vi "Add Point.vi"(8 "error in (no error)":errorcluster, 9 "Y":dbl, 10 "X":dbl, 11 "IV_data in":refnum<class "IV_data.lvclass">) -> (0 "error out":errorcluster, 3 "IV_data out":refnum<class "IV_data.lvclass">)   [LabVIEW 2014, in "IV_data.lvclass"]
uses:
  IV_data.lvclass
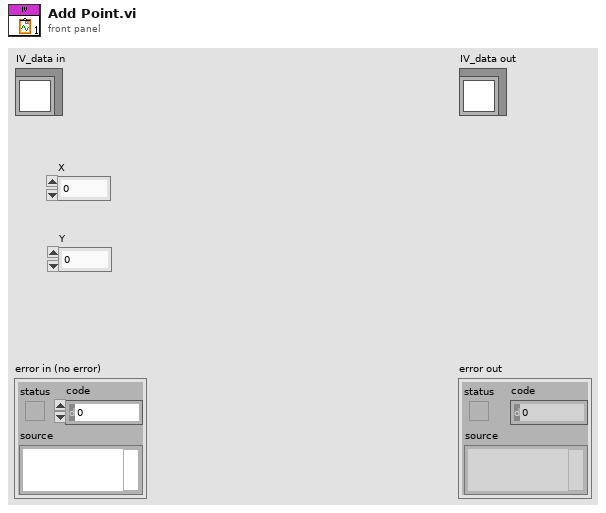
[diagram p1: front panel]
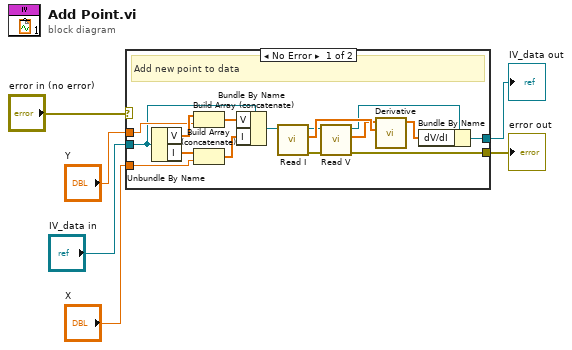
[diagram p0: block diagram]
diagram:
  n1 = case shown="No Error" "error in (no error)" {
    selector: "error in (no error)" -> [_ w23]
    tunnel: [w10 w23] -> w6
    tunnel: "Y" -> [w17 _]
    tunnel: "X" -> [w16 _]
    tunnel: "IV_data in" -> [w15 w24]
    tunnel: [w8 w24] -> w2
    frame No Error {
      # "Add new point to data"
      n2 = Unbundle By Name(w15) -> ("V"=w21:dbl[], "I"=w20:dbl[])
      n3 = Build Array (concatenate)(w21, w17) -> (w18:dbl[])
      n4 = Build Array (concatenate)(w20, w16) -> (w19:dbl[])
      n5 = Bundle By Name(cluster=w15, "V"=w18, "I"=w19) -> (w7:refnum<class "IV_data.lvclass">)
      n6 = call "Read I.vi"("IV_data in"=w7) -> ("error out"=w12:errorcluster, "I"=w14:dbl[], "IV_data out"=w13:refnum<class "IV_data.lvclass">)  [unwired: 8 in]
      n7 = call "Read V.vi"("error in (no error)"=w12, "IV_data in"=w13) -> ("error out"=w10:errorcluster, "V"=w11:dbl[], "IV_data out"=w9:refnum<class "IV_data.lvclass">)  [unwired: 7 in]
      n8 = call "Derivative.vi"("X"=w14, "Y"=w11) -> ("dY/dX"=w22:dbl[])  [unwired: 9 in]
      n9 = Bundle By Name(cluster=w9, "dV/dI"=w22) -> (w8:refnum<class "IV_data.lvclass">)
    }
    frame Error {
    }
  }
  "error out" <- w6
  "IV_data out" <- w2
